vi "benchmark-jitter.vi"(10 "wait (s)":dbl=0.001, 11 "iterations":i32=1000000) -> ()   [LabVIEW 2020]
panel:
  out "wfmg":dbl[][](graph)
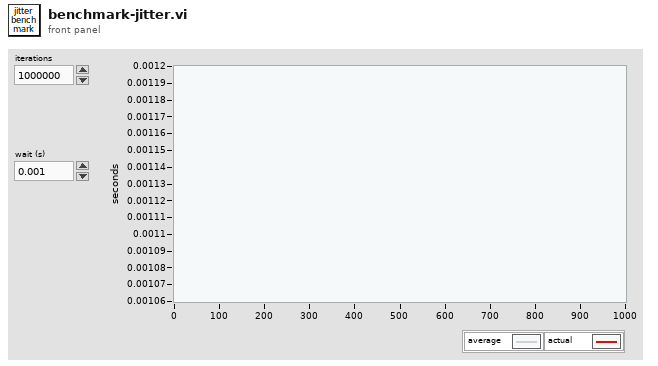
[diagram p1: front panel]
types:
  T1 = typedef "metadata.ctl" = cluster{"worker ID":u32, "min (s)":dbl, "max (s)":dbl, "mean (s)":dbl, "duration (s)":dbl}
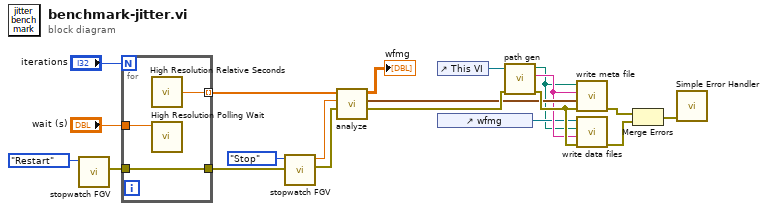
[diagram p0: block diagram]
diagram:
  n1 = call "stopwatch FGV.vi"("state"=enum16{"Restart", "Stop"}."Restart") -> ("error out"=w17:errorcluster)  [unwired: 9 in, 1 out]
  n2 = for {
    N: "iterations" -> [_]
    tunnel: "wait (s)" -> [w23]
    tunnel: [w22] -> w3 mode=indexing
    tunnel: w17 -> [w21]
    tunnel: [w21] -> w15
    n3 = call <vilib>:"High Resolution Relative Seconds.vi"() -> ("relative seconds"=w22:dbl)
    n4 = call <vilib>:"High Resolution Polling Wait.vi"("seconds to wait"=w23) -> ()  [unwired: 10 in, 1 out]
  }
  n5 = call "stopwatch FGV.vi"("error in"=w15, "state"=enum16{"Restart", "Stop"}."Stop") -> ("error out"=w1:errorcluster, "duration (s)"=w2:dbl)  [unwired: 8 in]
  n6 = call "analyze.vi"("error in"=w1, "duration (s)"=w2, "relative seconds"=w3) -> ("error out"=w13:errorcluster, "metadata"=w12:T1, "data"=→"wfmg":dbl[][])  [unwired: 6 in]
  n7 = control-ref of="This VI"() -> (w11:refnum<vi>)
  n8 = control-ref of="wfmg"() -> (w8:refnum<vi>)
  n9 = call "path gen.vi"("error in"=w13, "Calling VI"=w11) -> ("error out"=w14:errorcluster, "basename"=w9:string, "output folder"=w5:path)  [unwired: 7 in]
  n10 = call "write meta file.vi"("error in"=w14, "metadata"=w12, "file basename"=w9, "output folder"=w5) -> ("error out"=w7:errorcluster)  [unwired: 7 in]
  n11 = call "write data files.vi"("error in"=w14, "file basename"=w9, "output folder"=w5, "WaveformGraph in"=w8) -> ("error out"=w6:errorcluster)  [unwired: 7 in]
  n12 = Merge Errors(w7, w6) -> (w4:errorcluster)
  n13 = call <vilib>:"Simple Error Handler.vi"("error in (no error)"=w4) -> ()  [unwired: 4 in, 5 out]
